vi "GetDeviceList.vi"(7 "User":string="admin", 8 "error in (no error)":errorcluster, 11 "IcmMessageService in":refnum<class "IcmMessageService.lvclass">) -> (0 "IcmMessageService in 2":refnum<class "IcmMessageService.lvclass">, 2 "DeviceNames":string[](array[string]), 3 "DeviceList":T1[](array[typedef]))   [LabVIEW 2017]
uses:
  <vilib>/addons/InsightCM/MessageBus/MessageLibrary/SysCfgDeployer/controls/SysCfgDeployPackageRequestBody.ctl
  <vilib>/addons/InsightCM/MessageBus/MessageService/IcmMessageService.lvclass
panel:
  out "error out":errorcluster
  out "BadDevices":T1[](array[typedef])
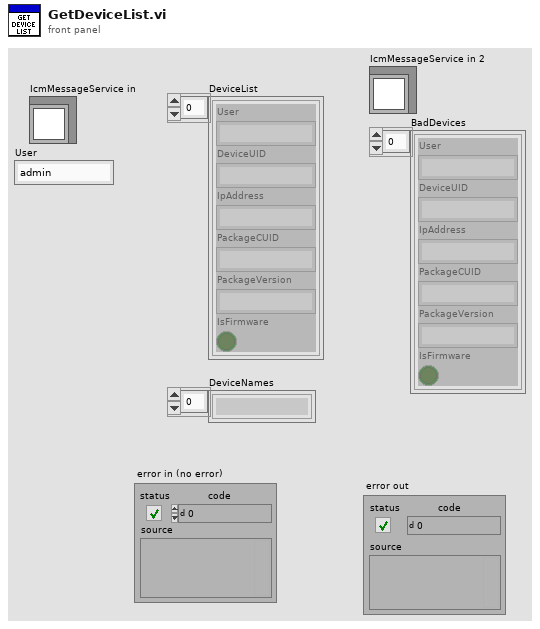
[diagram p1: front panel]
types:
  T1 = typedef "SysCfgDeployPackageRequestBody.ctl" = cluster{"User":string, "DeviceUID":string, "IpAddress":string, "PackageCUID":string, "PackageVersion":string, "IsFirmware":bool}
  T2 = typedef "AssetMgrGetDeviceListResponseBody.ctl" = cluster{"DeviceList":T3[]}
  T3 = typedef "Device.ctl" = cluster{"Id":string, "Name":string, "DeviceType":string, "HardwareName":string, "IpAddress":string, "HardwareInfo":T4[], "ApplicationType":string, "ApplicationVersion":string, "ConfigurationVersion":string, "State":T5, "Properties":T4[], "DataGroups":T6[], "BurstModeTrigger":T7}
  T4 = typedef "KeyValuePair.ctl" = cluster{"Key":string, "Value":string}
  T5 = typedef "DeviceState.ctl" = cluster{"Disabled":bool}
  T6 = typedef "DataGroup.ctl" = cluster{"Name":string, "AssetNodeId":string}
  T7 = typedef "BurstModeTrigger.ctl" = cluster{"Trigger":T8, "SampleRate":string, "AcquisitionLength":string}
  T8 = typedef "Trigger.ctl" = cluster{"Type":string, "Expression":string, "Conditions":T9[]}
  T9 = typedef "Condition.ctl" = cluster{"Source":string, "Type":string, "Operator":string, "CompareTo":string, "DwellSeconds":dbl}
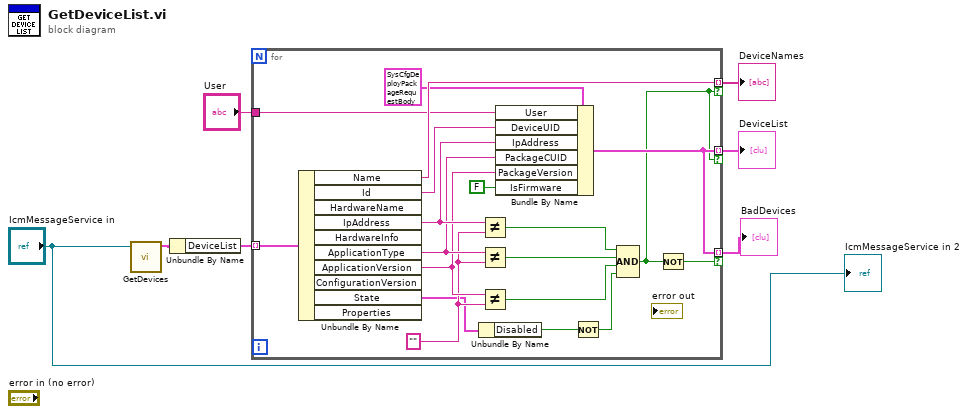
[diagram p0: block diagram]
diagram:
  n1 = call "GetDevices.vi"("service"="IcmMessageService in") -> ("Body"=w3:T2)  [unwired: 9 in, 1 out]
  n2 = Unbundle By Name(w3) -> ("DeviceList"=w4:T3[])
  n3 = for {
    tunnel: w4 -> [w26] mode=indexing
    tunnel: [w25] -> w5 mode=indexing if=w10
    tunnel: [w11] -> w7 mode=indexing if=w10
    tunnel: [w11] -> w2 mode=indexing if=w9
    tunnel: "User" -> [w8]
    w15 = "" ("y")
    n4 = Unbundle By Name(w26) -> ("Name"=w25:string, "Id"=w22:string, "IpAddress"=w21:string, "ApplicationType"=w20:string, "ApplicationVersion"=w16:string, "State"=w14:T5)  [unwired: 4 out]
    n5 = Unbundle By Name(w14) -> ("Disabled"=w13:bool)
    n6 = Not Equal?(x=w21, y=w15) -> (x != y?=w19:bool)
    n7 = Not Equal?(x=w20, y=w15) -> (x != y?=w18:bool)
    n8 = Not Equal?(x=w16, y=w15) -> (x != y?=w17:bool)
    n9 = Bundle By Name(cluster=T1 {"User"="admin", "DeviceUID"="5a21d8598e41741534c2e11d", "IpAddress"="10.2.104.72", "PackageCUID"="{F123D87A-D66C-9202-3ED6-47828FC48328}", "PackageVersion"="3.1.0", "IsFirmware"=FALSE} ("SysCfgDeployPackageRequest"), "User"=w8, "DeviceUID"=w22, "IpAddress"=w21, "PackageCUID"=w20, "PackageVersion"=w16, "IsFirmware"=FALSE) -> (w11:T1)
    n10 = Not(x=w13) -> (.not. x?=w12:bool)
    n11 = Compound Arithmetic op=AND(w19, w18, w17, w12) -> (w10:bool)
    n12 = Not(x=w10) -> (.not. x?=w9:bool)
  }
  "DeviceList" <- w7
  "DeviceNames" <- w5
  "BadDevices" <- w2
  "IcmMessageService in 2" <- "IcmMessageService in"
